vi "delay_sorter.vi"(0 "Out1 1":bool, 1 "Out1 2":bool, 5 "Out1 3":bool, 7 "Out1 4":bool, 9 "Out1 5":bool, 11 "Out1 6":bool, 12 "Out1 7":bool) -> (4 "Delay1":bool)   [LabVIEW 2013]
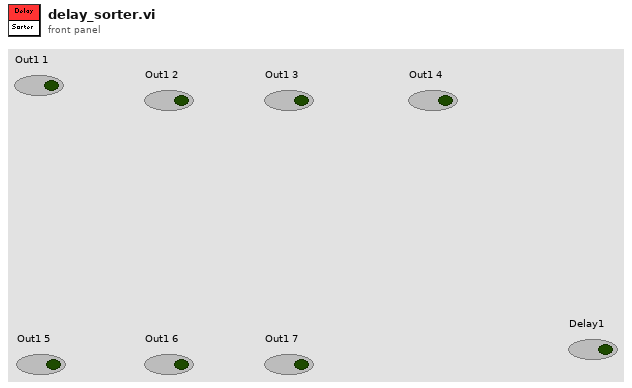
[diagram p1: front panel]
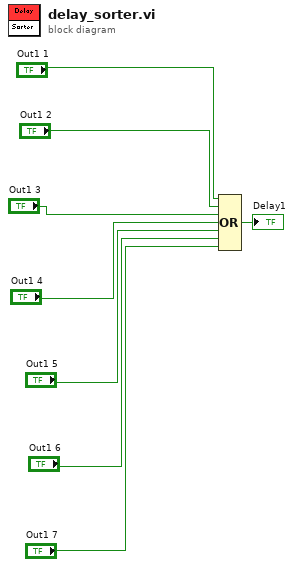
[diagram p0: block diagram]
diagram:
  n1 = Compound Arithmetic op=OR("Out1 1", "Out1 2", "Out1 3", "Out1 4", "Out1 5", "Out1 6", "Out1 7") -> (→"Delay1":bool)
